vi "Read String.vi"(8 "error in (no error)":errorcluster, 11 "Clock Time in":refnum<class "Clock Time.lvclass">) -> (0 "error out":errorcluster, 1 "Bytes Read":i32, 2 "String Read":string, 3 "Clock Time out":refnum<class "Clock Time.lvclass">)   [LabVIEW 2018, in "Clock Time.lvclass"]
doc: "Clock Timel.lvclass:Read String.vi\n\nThis VI reads the a string of data from the computer clock.\n\nInstrument Communication Module Version 1.0\nAugust, 2017 Original Code Consulting David Thomson\n www.originalcode.com"
uses:
  Clock Time.lvclass
  Clock Time.lvclass/Clock Time.ctl
panel:
  out "String Read":string
  out "String Read":string
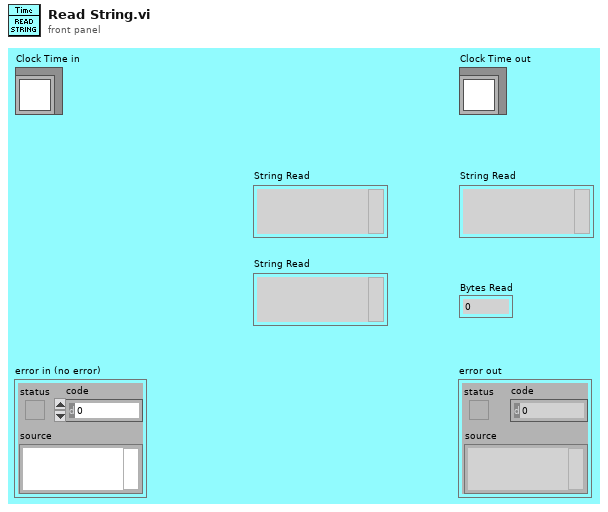
[diagram p1: front panel]
types:
  T1 = typedef "LVDateTimeRec.ctl" = cluster{"fractional second":dbl, "second":i32, "minute":i32, "hour":i32, "day of month":i32, "month":i32, "year":i32, "day of week":i32, "day of year":i32, "DST":i32}
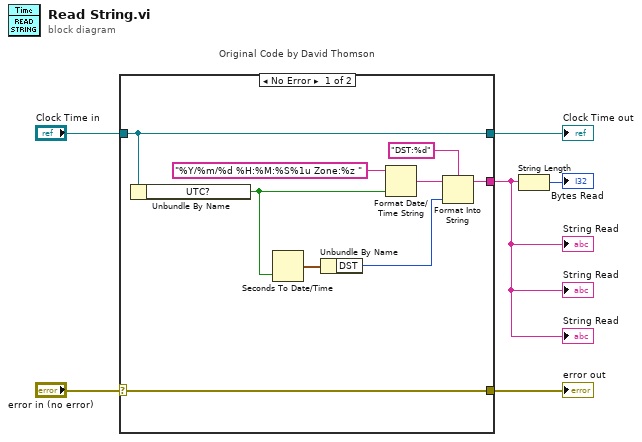
[diagram p0: block diagram]
diagram:
  n1 = case "Original Code by David Thomson" shown="No Error" "error in (no error)" {
    selector: "error in (no error)" -> [w13 w17]
    tunnel: [w13 w17] -> w5
    tunnel: [w14 w16] -> w3
    tunnel: "Clock Time in" -> [w14 w16]
    tunnel: [w9 _] -> w1
    frame No Error {
      n2 = Unbundle By Name(w14) -> ("UTC?"=w11:bool)
      n3 = Seconds To Date/Time(to UTC (F)=w11) -> (date time rec=w12:T1)  [unwired: 1 in]
      n4 = Unbundle By Name(w12) -> ("DST"=w7:i32)
      n5 = Format Date/Time String(time format string (%c)="%Y/%m/%d %H:%M:%S%1u Zone:%z ", UTC format=w11) -> (date/time string=w10:string)  [unwired: 1 out]
      n6 = Format Into String(format string="DST:%d", initial string=w10, w7) -> (resulting string=w9:string)  [unwired: 1 in, 1 out]
    }
    frame Error {
    }
  }
  "error out" <- w5
  "Clock Time out" <- w3
  "String Read" <- w1
  "String Read" <- w1
  "String Read" <- w1
  n7 = String Length(string=w1) -> (length=→"Bytes Read":i32)
